vi "open_app_ref.vi"(10 "timeout_ms":i32=60000, 11 "port":u16=3363) -> (3 "app_ref":u32)   [LabVIEW 2024]
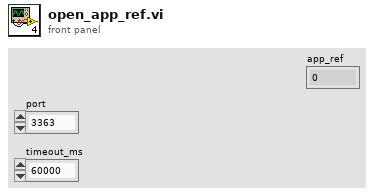
[diagram p1: front panel]
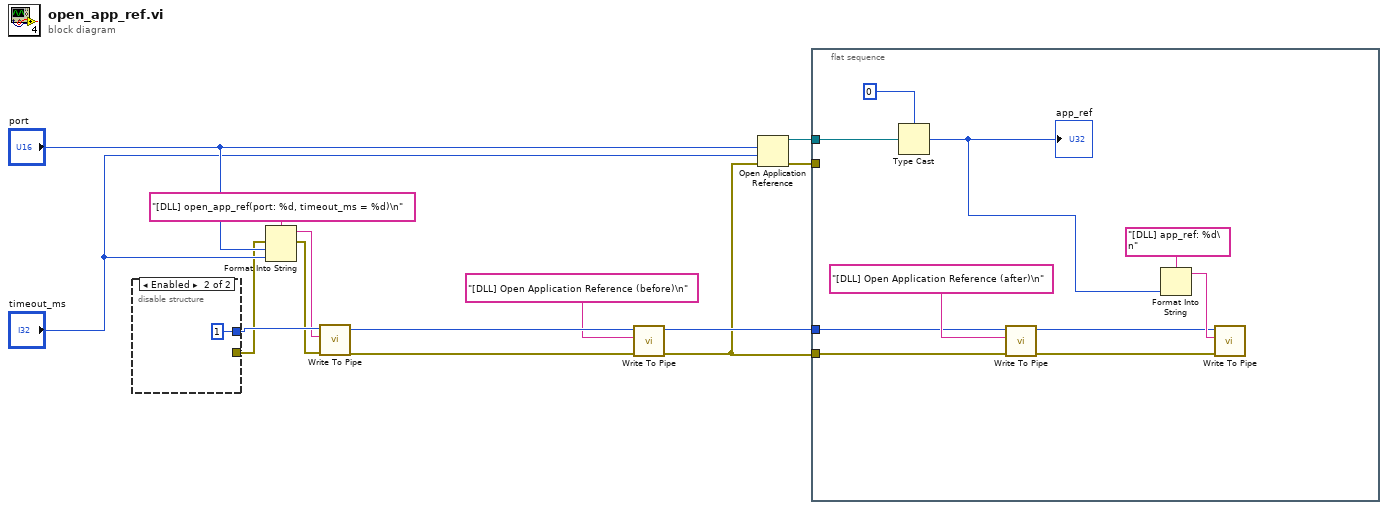
[diagram p0: block diagram]
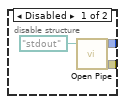
[diagram p2: hidden frame]
diagram:
  n1 = disable-structure shown="Enabled" {
    disable-tunnel: [w16 1 ("file descriptor")] -> w13
    disable-tunnel: [w15 _] -> w9
    frame Disabled {
      n2 = call <vilib>:"Open Pipe.vi"("path to named pipe"=path "stdout") -> ("error out"=w15:errorcluster, "file descriptor"=w16:i32)  [unwired: 3 in]
    }
    frame Enabled {
    }
  }
  n3 = Format Into String(format string="[DLL] open_app_ref(port: %d, timeout_ms = %d)\n", error in=w9, "port", "timeout_ms") -> (resulting string=w7:string, error out=w8:errorcluster)  [unwired: 1 in]
  n4 = call <vilib>:"Write To Pipe.vi"("error in (no error)"=w8, "data"=w7, "file descriptor"=w13) -> ("error out"=w4:errorcluster, "file descriptor"=w6:i32)  [unwired: 2 in, 1 out]
  n5 = call <vilib>:"Write To Pipe.vi"("error in (no error)"=w4, "data"="[DLL] Open Application Reference (before)\n" ("format string"), "file descriptor"=w6) -> ("error out"=w2:errorcluster, "file descriptor"=w3:i32)  [unwired: 2 in, 1 out]
  n6 = Open Application Reference(8:w2, 9:"timeout_ms", 10:"port") -> (0:w1:errorcluster, 3:w14:refnum<vi>)  [unwired: 1 in]
  n7 = flat-sequence {
    tunnel: w14 -> [w28]
    tunnel: w3 -> [w25]
    tunnel: w2 -> [w19]
    tunnel: w1 -> [_]
    frame #0 {
      n8 = Type Cast(type=u32 0, x=w28) -> (*(type *) &x=w22:u32)
      "app_ref" <- w22
      n9 = call <vilib>:"Write To Pipe.vi"("error in (no error)"=w19, "data"="[DLL] Open Application Reference (after)\n" ("format string"), "file descriptor"=w25) -> ("error out"=w21:errorcluster, "file descriptor"=w20:i32)  [unwired: 2 in, 1 out]
      n10 = Format Into String(format string="[DLL] app_ref: %d\n", w22) -> (resulting string=w23:string)  [unwired: 2 in, 1 out]
      n11 = call <vilib>:"Write To Pipe.vi"("error in (no error)"=w21, "data"=w23, "file descriptor"=w20) -> ()  [unwired: 2 in, 3 out]
    }
  }
